vi "Line sensor check.vi"() -> ()   [LabVIEW 2018]
doc: "The myRIO Project template acquires acceleration data from the onboard accelerometer and displays the changes of acceleration values in a waveform chart."
uses:
  Underlying VI's/Line Sensor AE/Line Sensor AE Type Def.ctl
panel:
  out "Line Sensor Raw Values":T1
  out "Line Detected?":bool
  in  "Stop Button":bool
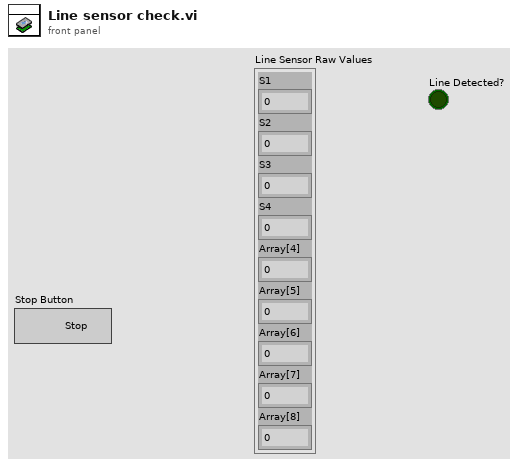
[diagram p1: front panel]
types:
  T1 = cluster{"S1":dbl, "S2":dbl, "S3":dbl, "S4":dbl, "Array[4]":dbl, "Array[5]":dbl, "Array[6]":dbl, "Array[7]":dbl, "Array[8]":dbl}
  T2 = typedef "Line Sensor AE Type Def.ctl" = enum16{"INIT AE", "READ FROM LINE SENSORS"}
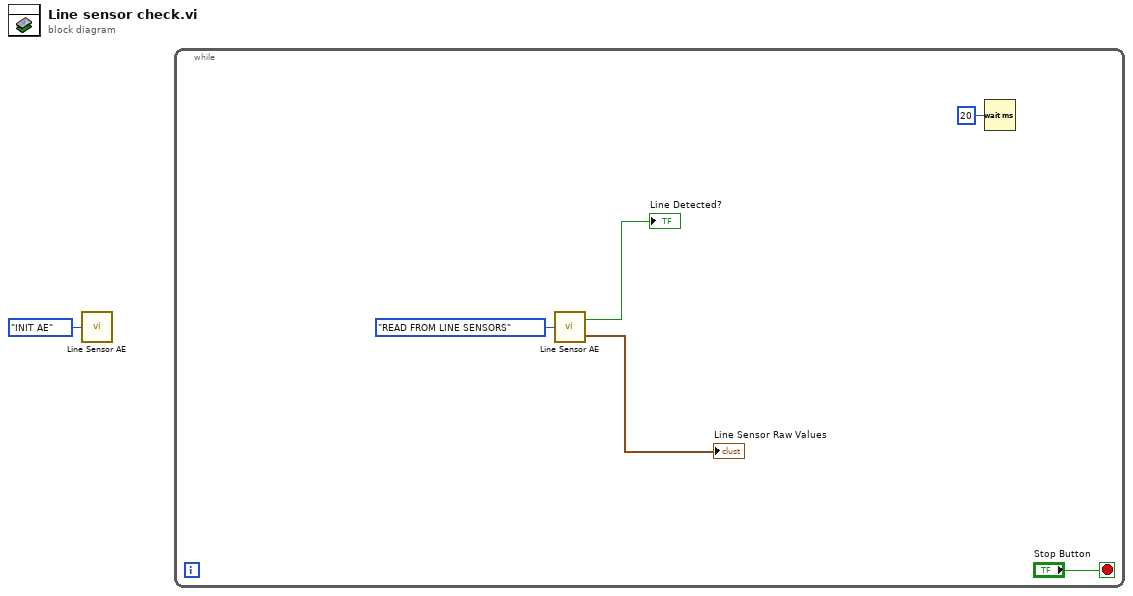
[diagram p0: block diagram]
diagram:
  n1 = call "Line Sensor AE.vi"("AE State"=Line_Sensor_AE_Type_Def."INIT AE") -> ()  [unwired: 2 out]
  n2 = while {
    stop <- "Stop Button" stop-if-true
    n3 = call "Line Sensor AE.vi"("AE State"=Line_Sensor_AE_Type_Def."READ FROM LINE SENSORS") -> ("Line Detected?"=→"Line Detected?":bool, "Line Sensor Raw Values"=→"Line Sensor Raw Values":T1)
    n4 = Wait (ms)(milliseconds to wait=u32 20) -> ()  [unwired: 1 out]
  }
